vi "RunLogRecordDynamic.vi"(8 "error in (no error)":errorcluster, 11 "Config":T1={"LogName"="", "Level"=enum."Info", "LogFolder"=path "", "MaxFileSize"=0, "FileExtension"="", "TimeSytle"="", "LogStyle"=""}) -> (0 "error out":errorcluster)   [LabVIEW 2016, in "Log4Lv.lvlib"]
doc: "Use this template to build a VI to use as a subVI."
uses:
  Log4Lv.lvlib
  RunLogRecord.vi
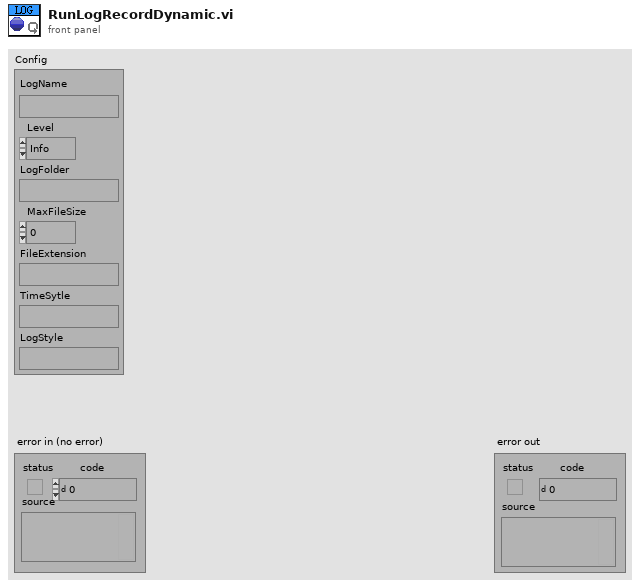
[diagram p1: front panel]
types:
  T1 = cluster{"LogName":string, "Level":enum16{"Disable", "Error", "Warn", "Info", "Debug"}, "LogFolder":path, "MaxFileSize":i32, "FileExtension":string, "TimeSytle":string, "LogStyle":string}
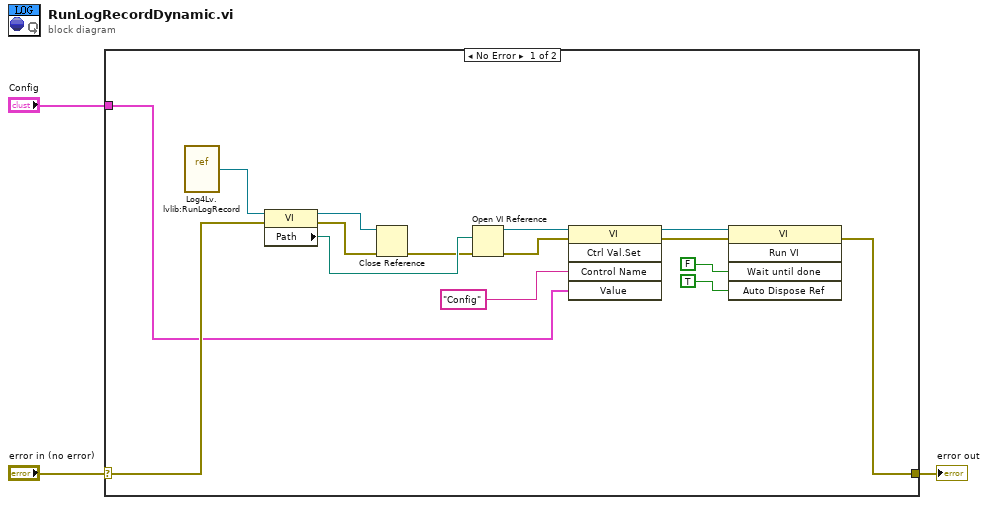
[diagram p0: block diagram]
diagram:
  n1 = case shown="No Error" "error in (no error)" {
    selector: "error in (no error)" -> [w6 w19]
    tunnel: [w5 w19] -> w2
    tunnel: "Config" -> [w4 _]
    frame No Error {
      n2 = vi-ref "Log4Lv.lvlib:RunLogRecord.vi"() -> (w7:refnum<vi>)
      n3 = property class="VI"(reference=w7, error in=w6) -> (reference out=w13:refnum<vi>, error out=w18:errorcluster, "Path"=w17:path)
      n4 = Close Reference(reference=w13, error in (no error)=w18) -> (error out=w14:errorcluster)
      n5 = Open VI Reference(vi path=w17, error in (no error)=w14) -> (vi reference=w12:refnum<vi>, error out=w10:errorcluster)  [unwired: 4 in]
      n6 = invoke class="VI" method="Ctrl Val.Set"(reference=w12, error in=w10, "Control Name"="Config", "Value"=w4) -> (reference out=w11:refnum<vi>, error out=w9:errorcluster)  [unwired: 1 in, 3 out]
      n7 = invoke class="VI" method="Run VI"(reference=w11, error in=w9, "Wait until done"=FALSE ("Wait Until Done"), "Auto Dispose Ref"=TRUE ("Auto Dispose Reference")) -> (error out=w5:errorcluster)  [unwired: 1 in, 4 out]
    }
    frame Error {
    }
  }
  "error out" <- w2
